vi "StageReadPos.vi"(8 "error in (no error)":errorcluster, 10 "Stage Select":T1, 11 "Device In":T2) -> (0 "error out":errorcluster, 3 "CurrentPosition":dbl)   [LabVIEW 2014]
doc: "Read the current stage position"
uses:
  C:/Users/light/Desktop/SI+Raman/Labview/Raman/dll/ThorLabs.MotionControl.KCube.DCServoCLI.dll
  dll/ThorLabs.MotionControl.KCube.DCServoCLI.dll
  TypeDef/StageDeviceOut.ctl
  TypeDef/StageSelect.ctl
panel:
  # "Read the current stage position"
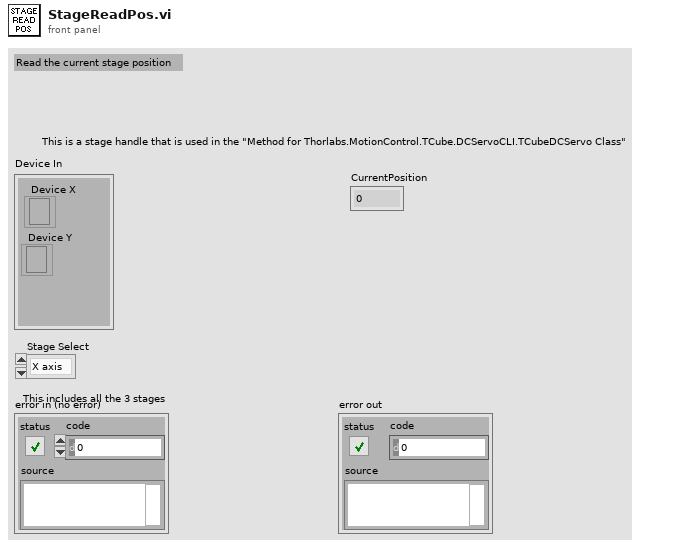
[diagram p1: front panel]
types:
  T1 = typedef "StageSelect.ctl" = enum16{"X axis", "Y axis", "Z axis"}
  T2 = typedef "StageDeviceOut.ctl" = cluster{"Device X":refnum<k24>, "Device Y":refnum<k24>}
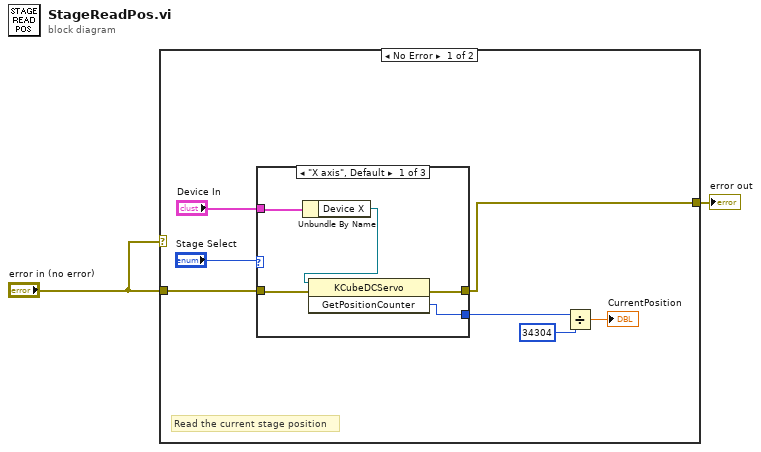
[diagram p0: block diagram]
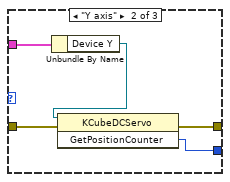
[diagram p2: hidden frame]
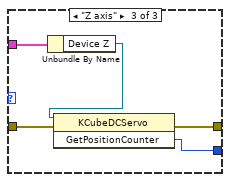
[diagram p3: hidden frame]
diagram:
  n1 = case shown="No Error" "error in (no error)" {
    tunnel: "error in (no error)" -> [w7 w25]
    tunnel: [w5 w25] -> w1
    frame No Error {
      # "Read the current stage position"
      n2 = case shown="\"X axis\", Default" "Stage Select" {
        tunnel: w7 -> [w12 w19 w22]
        tunnel: [w11 w18 w21] -> w5
        tunnel: [w10 w17 w20] -> w4
        tunnel: "Device In" -> [w13 w16 w23]
        frame "X axis", Default {
          n3 = Unbundle By Name(w13) -> ("Device X"=w14:refnum<k24>)
          n4 = invoke class="KCubeDCServo" method="GetPositionCounter"(reference=w14, error in=w12) -> (error out=w11:errorcluster, "GetPositionCounter"=w10:i32)  [unwired: 1 in, 1 out]
        }
        frame "Y axis" {
          n5 = Unbundle By Name(w16) -> ("Device Y"=w15:refnum<k24>)
          n6 = invoke class="KCubeDCServo" method="GetPositionCounter"(reference=w15, error in=w19) -> (error out=w18:errorcluster, "GetPositionCounter"=w17:i32)  [unwired: 1 in, 1 out]
        }
        frame "Z axis" {
          n7 = Unbundle By Name(w23) -> ("Device Z"=w24:refnum<k24>)
          n8 = invoke class="KCubeDCServo" method="GetPositionCounter"(reference=w24, error in=w22) -> (error out=w21:errorcluster, "GetPositionCounter"=w20:i32)  [unwired: 1 in, 1 out]
        }
      }
      n9 = Divide(x=w4, y=34304) -> (x/y=→"CurrentPosition":dbl)
    }
    frame Error {
    }
  }
  "error out" <- w1
